vi "Create From EventStructure Reference.vi"(8 "error in (no error)":errorcluster, 11 "CaseStructure":refnum<vi>) -> (0 "error out":errorcluster, 3 "CSM-Helper.lvclass":refnum<class "CSM-Helper.lvclass">)   [LabVIEW 2017, in "CSM-Helper.lvclass"]
doc: "### Create From EventStructure Reference.vi\n\n-- <b>Controls</b> --\n- <b>CaseStructure</b>:\n\n-- <b>Indicators</b> --\n- <b>CSM-Helper.lvclass</b>:"
uses:
  CSM-Helper.lvclass
  CSM-Helper.lvclass/CSM-Helper.ctl
  Utility/CSM-Helper Utility.lvlib
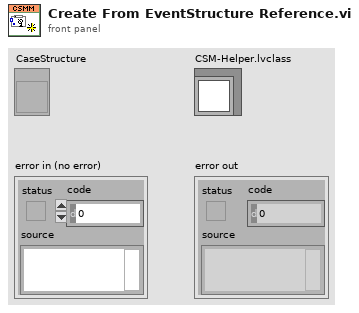
[diagram p1: front panel]
types:
  T1 = typedef "CSM-Helper Utility.lvlib/CSM Basic Refs.ctl" = cluster{"VI":refnum<vi>, "While Loop":refnum<vi>, "Case Structure":refnum<vi>, "Parse State Queue":refnum<vi>, "Event Structure":refnum<vi>, "Type":T2, "InLvlibp":bool}
  T2 = typedef "CSM-Helper Utility.lvlib/CSM Module Type.ctl" = enum16{"Not a CSM", "JKISM", "CSM"}
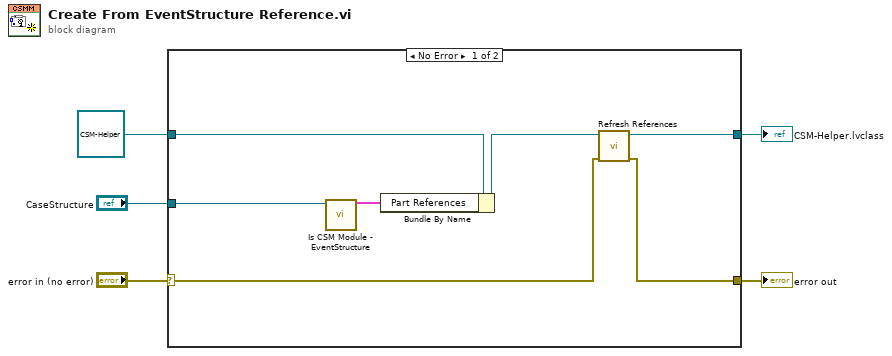
[diagram p0: block diagram]
diagram:
  n1 = case shown="No Error" "error in (no error)" {
    selector: "error in (no error)" -> [w6 w14]
    tunnel: [w9 w14] -> w4
    tunnel: [w10 w13] -> w2
    tunnel: refnum<class "CSM-Helper.lvclass"> refnum ("JKI SM") -> [w12 w13]
    tunnel: "CaseStructure" -> [w7 _]
    frame No Error {
      n2 = call "Is CSM Module - EventStructure.vi"("EventStructure"=w7) -> ("CSM Basic Refs"=w8:T1)  [unwired: 8 in, 2 out]
      n3 = Bundle By Name(cluster=w12, "Part References"=w8) -> (w11:refnum<class "CSM-Helper.lvclass">)
      n4 = call "Refresh References.vi"("error in (no error)"=w6, "CSM-Helper in"=w11) -> ("error out"=w9:errorcluster, "CSM-Helper out"=w10:refnum<class "CSM-Helper.lvclass">)  [unwired: 8 in]
    }
    frame Error {
    }
  }
  "error out" <- w4
  "CSM-Helper.lvclass" <- w2
